vi "Function data mismatch error.vi"(8 "error in (no error)":errorcluster) -> (0 "error out":errorcluster)   [LabVIEW 2013, in "Modbus Library - Advance.lvlib" / "Master Function Definition.lvclass"]
doc: "Throws error when called. This error should be used to indicate that the returned data (ie for write functions) does not match the data sent."
uses:
  Master Function Definition.lvclass
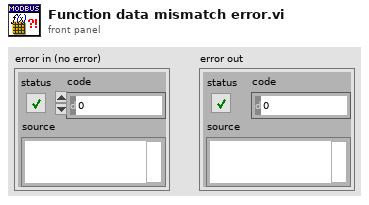
[diagram p1: front panel]
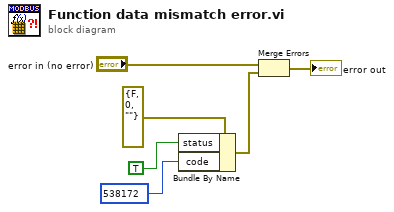
[diagram p0: block diagram]
diagram:
  n1 = Bundle By Name(cluster=errorcluster {"status"=FALSE, "code"=0, "source"=""} ("error constant"), "status"=TRUE, "code"=538172) -> (w3:errorcluster)
  n2 = Merge Errors("error in (no error)", w3) -> (→"error out":errorcluster)
